vi "Temp Value Changed.vi"(8 "error in (no error)":errorcluster, 10 "Current Temp. Value":dbl, 11 "Central Control in":refnum<class "Central Control.lvclass">) -> (0 "error out":errorcluster, 3 "Central Control out":refnum<class "Central Control.lvclass">)   [LabVIEW 2021, in "Central Control.lvlib" / "Central Control.lvclass"]
uses:
  Central Control.lvclass
  Central Control.lvclass/Central Control.ctl
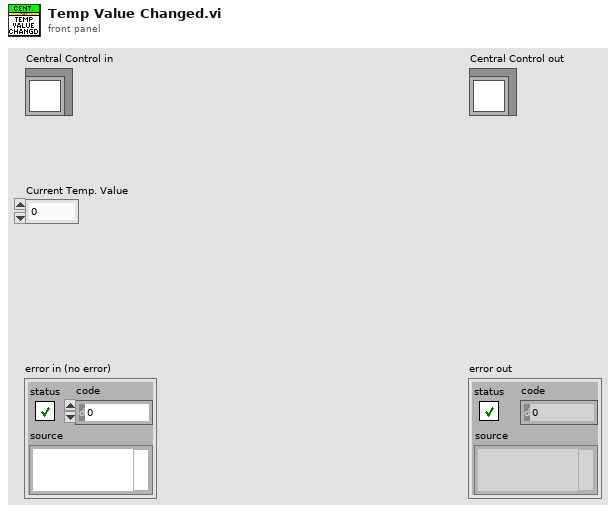
[diagram p1: front panel]
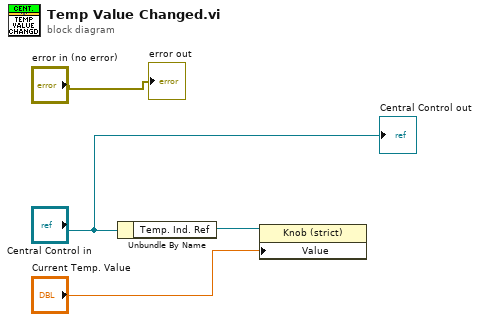
[diagram p0: block diagram]
diagram:
  n1 = Unbundle By Name("Central Control in") -> ("Temp. Ind. Ref"=w4:refnum<vi>)
  n2 = property class="Knob (strict)"(reference=w4, "Value"="Current Temp. Value") -> ()  [unwired: 1 in, 2 out]
  "error out" <- "error in (no error)"
  "Central Control out" <- "Central Control in"
